vi "Configure OCP.vi"(8 "error in (no error)":errorcluster, 9 "Current Limit (0.0 V)":dbl format="%.2g", 10 "Enable OCP (T: Enable)":bool=TRUE, 11 "VISA resource name":refnum<visa-resource-name>) -> (0 "error out":errorcluster, 3 "VISA resource name out":refnum<visa-resource-name>)   [LabVIEW 2013, in "IT6900.lvlib"]
doc: "Set current limit of current protection to <b>OCP</b>. If the peak value of the output current is higher than the OCP limit, the output of the power supply will turn off and alarm will be sent out"
uses:
  IT6900.lvlib
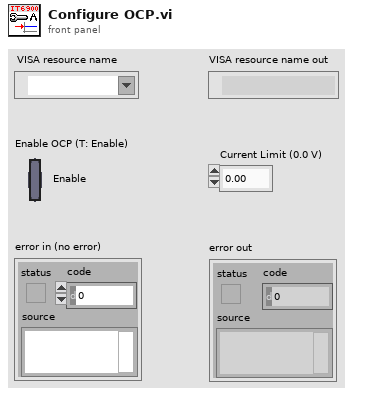
[diagram p1: front panel]
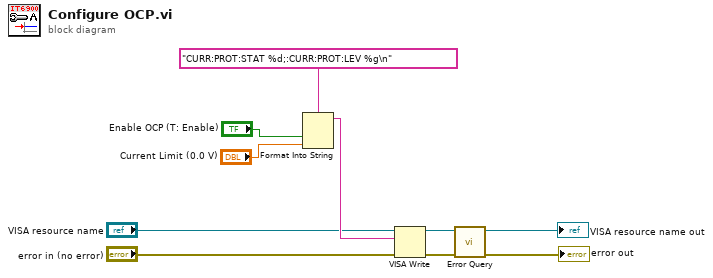
[diagram p0: block diagram]
diagram:
  n1 = Format Into String(format string="CURR:PROT:STAT %d;:CURR:PROT:LEV %g\n", "Enable OCP (T: Enable)", "Current Limit (0.0 V)") -> (resulting string=w7:string)  [unwired: 2 in, 1 out]
  n2 = VISA Write(VISA resource name="VISA resource name", write buffer=w7, error in (no error)="error in (no error)") -> (VISA resource name out=w3:refnum<visa-resource-name>, error out=w4:errorcluster)  [unwired: 1 out]
  n3 = call "Error Query.vi"("error in (no error)"=w4, "VISA resource name"=w3) -> ("error out"=→"error out":errorcluster, "VISA resource name out"=→"VISA resource name out":refnum<visa-resource-name>)  [unwired: 6 in, 2 out]
